vi "+S2C_FORNAX_Process.vi"(8 "Error In":errorcluster) -> (0 "Error Out":errorcluster)   [LabVIEW 2015]
uses:
  VIs/S2C_FORNAX_Proc_Globals.vi
panel:
  out "Err":bool
  out "Init":bool
  in  "Clear":bool
  out "Exit":bool
  in  "LogDepth":u32=500 caption="Log Depth"
  in  "CtrlTab":enum32{"Fornax", "Viper", "DDS Log"}(tab)
  in  "P1":T1 {"P1C1"."Return" items=["Partition", "Message", "M_BarcodeImageFile", "ErrorStatus"]; "P1C1"."Cmd" items=["BarcodeImageCommand", "BoardIdCommand", "Close", "DftAlarmCommand", "DftAudioPlayCommand", "DftInstrumentCommand", "DftLogCommand", "EmA2dCalDataCommand", "EnergyParameterCommand", "ExternalCommCommand", "FeatureSettingsCommand", "FornaxCommand", "General", "InstrumentSettingCommand", "Launch", "MonopolarCommand", "Open", "SupervisorCommand", "SwitchStatus", "SystemConfigurationCommand", "SystemSettingsCommand", "TimeCommand", "UserSettingsCommand", "ViperCmd", "VolumeBarsCommand"]}
  in  "P2":T2={"P2C1"={"VIP_Cmd"="", "VIP_RX"="", "VIP_Browse"=FALSE, "VIP_Send"=FALSE, "VIP_Clear"=FALSE, "VipLogDepth"=50, "VIP_Auto"=TRUE}}
  in  "P3":T3={"P3C1"={"DDS Log"="", "DDS_Clear"=FALSE, "DdsLogDepth"=1000, "DDS_Auto"=TRUE}}
  in  "CommLog":string caption="Communication Log"
  # "Main Cluster:\n394x886\n1 = 355x876\n2 = 355x438\n3 = 355x292\n4 = 163x438\n6 = 163x292\n8 = 163x219"
  # "Fornax Driver Panel"
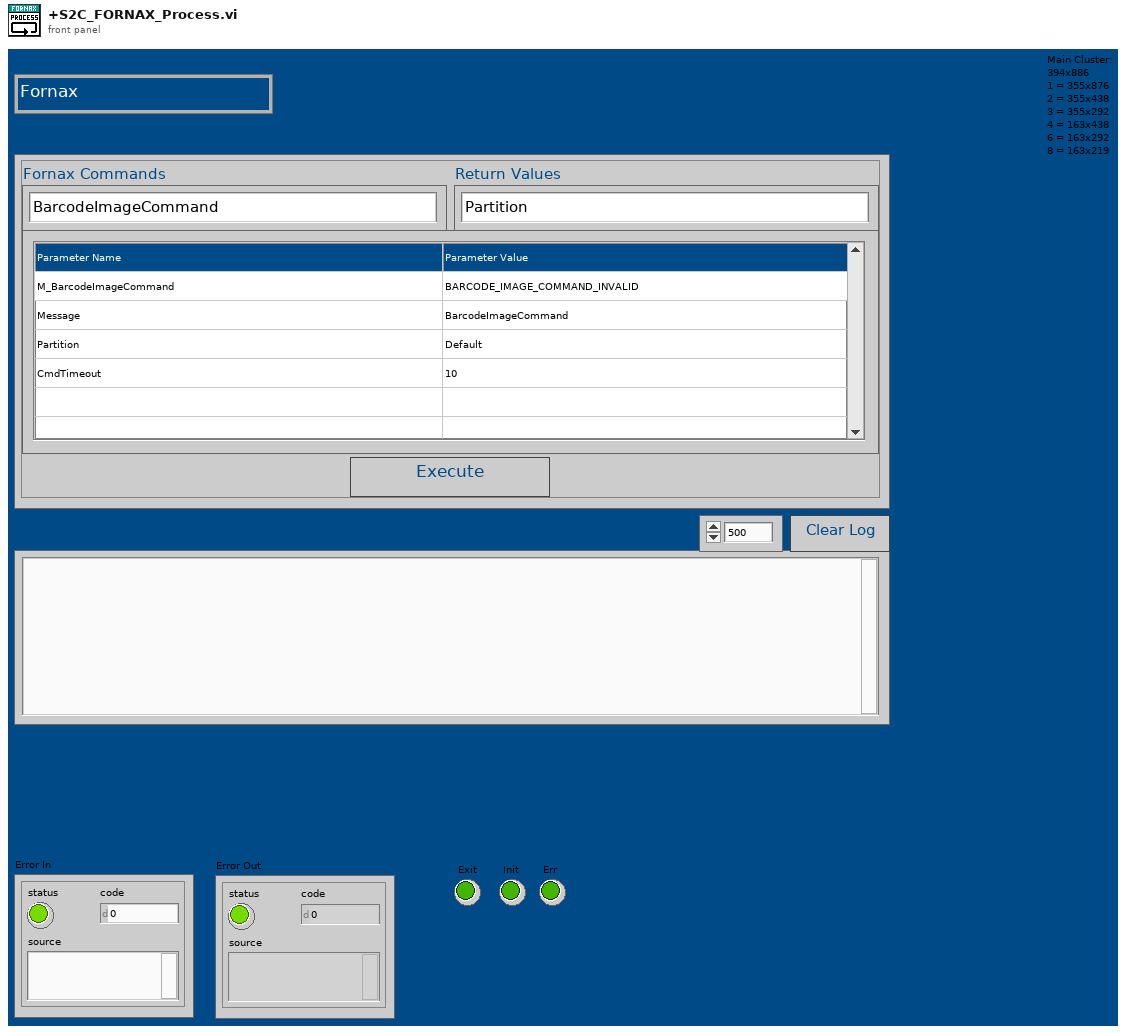
[diagram p1: front panel]
types:
  T1 = cluster{"P1C1":cluster{"P1C1Exe":bool, "Cmd":u16, "Return":u16, "Params":i32}}
  T2 = cluster{"P2C1":cluster{"VIP_Cmd":string, "VIP_RX":string, "VIP_Browse":bool, "VIP_Send":bool, "VIP_Clear":bool, "VipLogDepth":u32, "VIP_Auto":bool}}
  T3 = cluster{"P3C1":cluster{"DDS Log":string, "DDS_Clear":bool, "DdsLogDepth":u32, "DDS_Auto":bool}}
  T4 = cluster{"RawMsg":string, "ViperMsg":string[], "DDSMsg":string[]}
  T5 = typedef "LVPoint32TypeDef.ctl" = cluster{"Horizontal":i32, "Vertical":i32}
  T6 = typedef "LVRowAndColumnTypeDef.ctl" = cluster{"Row":i32, "Column":i32}
  T7 = cluster{"Caller-Q":refnum<queue>, "Command":string, "Return":string, "Data":variant, "Timeout":dbl}
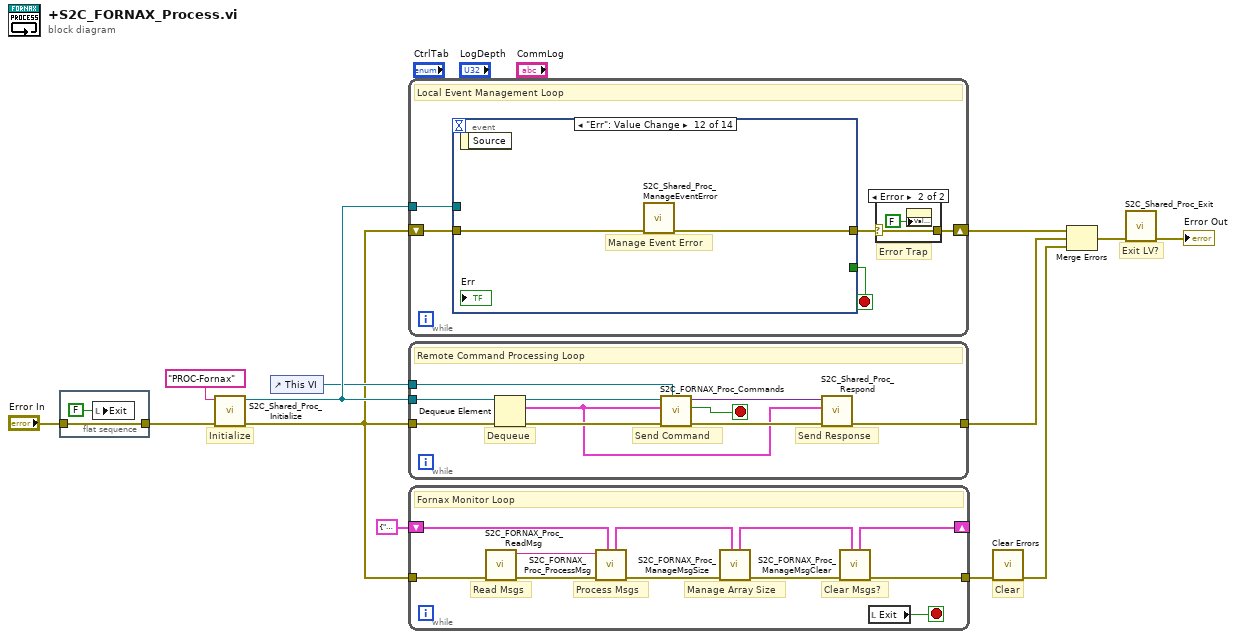
[diagram p0: block diagram]
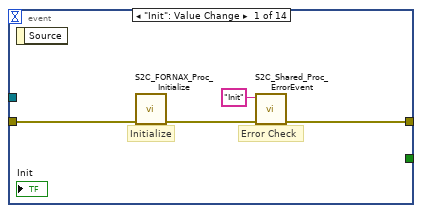
[diagram p3: hidden frame]
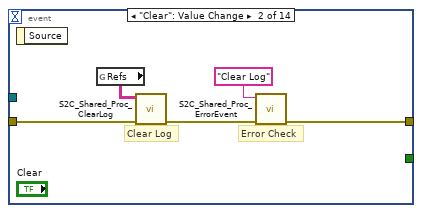
[diagram p4: hidden frame]
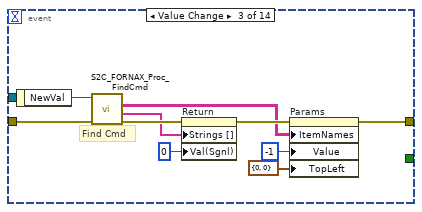
[diagram p5: hidden frame]
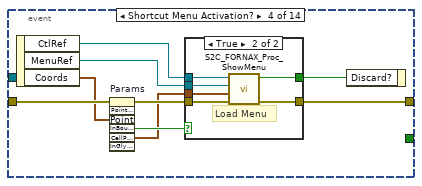
[diagram p6: hidden frame]
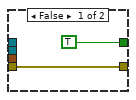
[diagram p7: hidden frame]
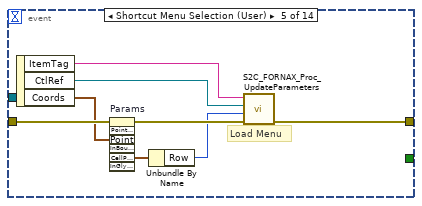
[diagram p8: hidden frame]
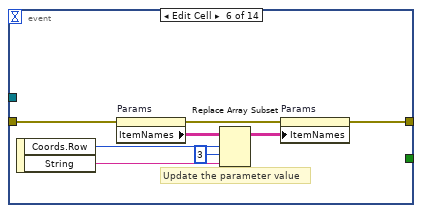
[diagram p9: hidden frame]
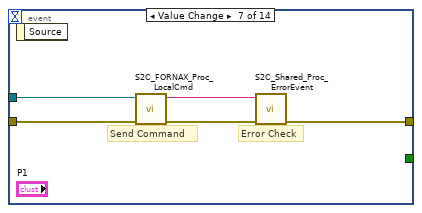
[diagram p10: hidden frame]
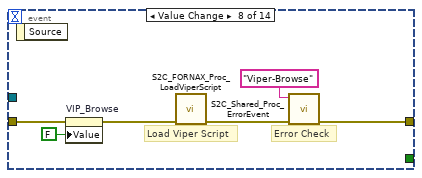
[diagram p11: hidden frame]
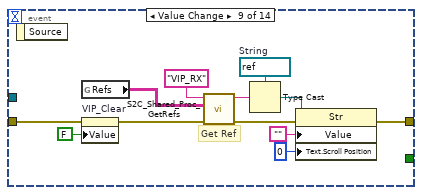
[diagram p12: hidden frame]
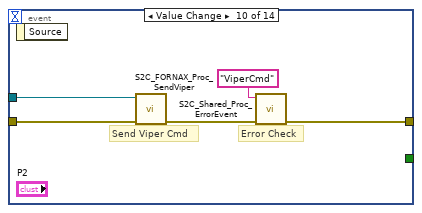
[diagram p13: hidden frame]
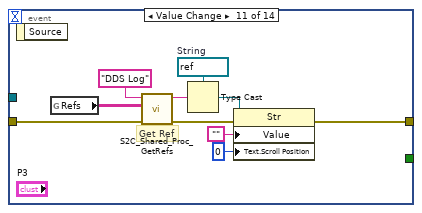
[diagram p14: hidden frame]
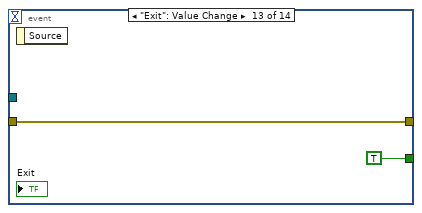
[diagram p15: hidden frame]
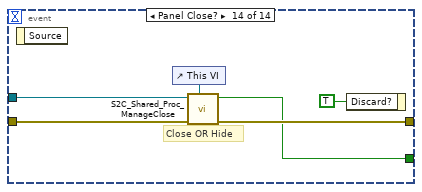
[diagram p16: hidden frame]
diagram:
  # "Clear"
  # "Exit LV?"
  # "Initialize"
  n1 = flat-sequence {
    tunnel: "Error In" -> [w14]
    tunnel: [w14] -> w1
    frame #0 {
      n2 = local write "Exit"(FALSE ("Exit?")) -> ()
    }
  }
  n3 = call "S2C_Shared_Proc_Initialize.vi"("Error In"=w1, "Q-Name"="PROC-Fornax" ("name (unnamed)")) -> ("Error Out"=w2:errorcluster, "Q-Ref"=w9:refnum<queue>)  [unwired: 8 in]
  n4 = control-ref of="This VI"() -> (w6:refnum<vi>)
  n5 = while {
    tunnel: w9 -> [w19]
    shift-right: [w16] -> w13
    shift-left: w2 -> [w20]
    stop <- w18 stop-if-true
    # "Error Trap"
    # "Local Event Management Loop"
    n6 = event shown="[11] \"Err\": Value Change" {
      selector: _ -> [_ _ _ _ _ _ _ _ _ _ _ _ _ _]
      dyn-events: _ -> [_ _ _ _ _ _ _ _ _ _ _ _ _ _]
      timeout: _ -> [_ _ _ _ _ _ _ _ _ _ _ _ _ _]
      tunnel: w20 -> [w27 w32 w42 w51 w67 w75 w79 w86 w89 w103 w106 w115 w117 w122]
      tunnel: w19 -> [_ _ _ _ _ _ w80 _ _ w102 _ _ _ w120]
      tunnel: [w25 w29 w36 w43 w62 w69 w77 w82 w90 w99 w105 w114 w117 w121] -> w17
      tunnel: [_ _ _ _ _ _ _ _ _ _ _ _ TRUE ("Discard?") w119] -> w18
      event "Init": Value Change {
        # "Error Check"
        # "Initialize"
        n7 = event-data() -> ()  [unwired: 1 in, 1 out]
        n8 = call "S2C_FORNAX_Proc_Initialize.vi"("Error In"=w27) -> ("Error Out"=w26:errorcluster)  [unwired: 10 in]
        n9 = call "S2C_Shared_Proc_ErrorEvent.vi"("Error In"=w26, "Command"="Init") -> ("Error Out"=w25:errorcluster)  [unwired: 9 in]
      }
      event "Clear": Value Change {
        # "Error Check"
        # "Clear Log"
        n10 = event-data() -> ()  [unwired: 1 in, 1 out]
        n11 = global read "S2C_FORNAX_Proc_Globals.vi" "Refs"() -> (w31:string[][])
        n12 = call "S2C_Shared_Proc_ClearLog.vi"("Error In"=w32, "Refs"=w31) -> ("Error Out"=w30:errorcluster)  [unwired: 9 in]
        n13 = call "S2C_Shared_Proc_ErrorEvent.vi"("Error In"=w30, "Command"="Clear Log") -> ("Error Out"=w29:errorcluster)  [unwired: 9 in]
      }
      event "P1.P1C1.Cmd": Value Change {
        # "Find Cmd"
        n14 = event-data() -> ("NewVal"=w41:u16)  [unwired: 1 in]
        n15 = call "S2C_FORNAX_Proc_FindCmd.vi"("Error In"=w42, "Index"=w41) -> ("Error Out"=w40:errorcluster, "Returns"=w39:string[], "Parameters"=w33:string[][])  [unwired: 6 in, 1 out]
        n16 = property on="Return" class="Ring (strict)"(error in=w40, "Strings []"=w39, "Val(Sgnl)"=u16 0 ("Value (Signaling)")) -> (error out=w37:errorcluster)  [unwired: 1 in, 1 out]
        n17 = property on="Params" class="MCListbox (strict)"(error in=w37, "ItemNames"=w33, "Value"=-1, "TopLeft"=cluster{"Row":u32, "Column":u32} {"Row"=0, "Column"=0} ("Top Left Visible Cell")) -> (error out=w36:errorcluster)  [unwired: 1 in, 1 out]
      }
      event "P1.P1C1.Params": Shortcut Menu Activation? {
        n18 = event-data() -> ("CtlRef"=w47:refnum<vi>, "MenuRef"=w46:refnum<k9>, "Coords"=w50:T5)  [unwired: 1 in]
        n19 = invoke on="Params" class="MCListbox (strict)" method="Point To Row Column"(error in=w51, "Point"=w50) -> (error out=w49:errorcluster, "InBounds"=w48:bool, "CellPosition"=w45:T6)  [unwired: 5 in, 4 out]
        n20 = case shown="True" w48 {
          tunnel: w49 -> [w53 w59]
          tunnel: w45 -> [_ w58]
          tunnel: w46 -> [_ w57]
          tunnel: w47 -> [_ w56]
          tunnel: [w53 w55] -> w43
          tunnel: [TRUE ("Discard?") w54] -> w44
          frame False {
          }
          frame True {
            # "Load Menu"
            n21 = call "S2C_FORNAX_Proc_ShowMenu.vi"("Error In"=w59, "Cell Position"=w58, "MenuRef"=w57, "CtlRef"=w56) -> ("Error Out"=w55:errorcluster, "Discard?"=w54:bool)  [unwired: 6 in]
          }
        }
        n22 = event-data("Discard?"=w44) -> ()  [unwired: 1 in, 1 out]
      }
      event "P1.P1C1.Params": Shortcut Menu Selection (User) {
        # "Load Menu"
        n23 = event-data() -> ("ItemTag"=w64:string, "CtlRef"=w63:refnum<vi>, "Coords"=w66:T5)  [unwired: 1 in]
        n24 = invoke on="Params" class="MCListbox (strict)" method="Point To Row Column"(error in=w67, "Point"=w66) -> (error out=w65:errorcluster, "CellPosition"=w61:T6)  [unwired: 5 in, 5 out]
        n25 = Unbundle By Name(w61) -> ("Row"=w60:i32)
        n26 = call "S2C_FORNAX_Proc_UpdateParameters.vi"("Error In"=w65, "Row"=w60, "CtlRef"=w63, "ItemTag"=w64) -> ("Error Out"=w62:errorcluster)  [unwired: 7 in]
      }
      event "P1.P1C1.Params": Edit Cell {
        # "Update the parameter value"
        n27 = event-data() -> ("Coords.Row"=w71:i32, "String"=w72:string)  [unwired: 1 in]
        n28 = property on="Params" class="MCListbox (strict)"(error in=w75) -> (error out=w70:errorcluster, "ItemNames"=w73:string[][])  [unwired: 1 in, 1 out]
        n29 = Replace Array Subset(array=w73, new element=w72, index (row)=w71, index (col)=3 ("disabled index (col)")) -> (w68:string[][])
        n30 = property on="Params" class="MCListbox (strict)"(error in=w70, "ItemNames"=w68) -> (error out=w69:errorcluster)  [unwired: 1 in, 1 out]
      }
      event "P1.P1C1.P1C1Exe": Value Change {
        # "Error Check"
        # "Send Command"
        n31 = event-data() -> ()  [unwired: 1 in, 1 out]
        n32 = call "S2C_FORNAX_Proc_LocalCmd.vi"("Error In"=w79, "Q-Ref"=w80) -> ("Error Out"=w78:errorcluster, "Command"=w76:string)  [unwired: 8 in]
        n33 = call "S2C_Shared_Proc_ErrorEvent.vi"("Error In"=w78, "Command"=w76) -> ("Error Out"=w77:errorcluster)  [unwired: 9 in]
      }
      event "P2.P2C1.VIP_Browse": Value Change {
        # "Error Check"
        # "Load Viper Script"
        n34 = event-data() -> ()  [unwired: 1 in, 1 out]
        n35 = property on="VIP_Browse" class="Bool (strict)"(error in=w86, "Value"=FALSE) -> (error out=w85:errorcluster)  [unwired: 1 in, 1 out]
        n36 = call "S2C_FORNAX_Proc_LoadViperScript.vi"("Error In"=w85) -> ("Error Out"=w83:errorcluster)  [unwired: 10 in]
        n37 = call "S2C_Shared_Proc_ErrorEvent.vi"("Error In"=w83, "Command"="Viper-Browse") -> ("Error Out"=w82:errorcluster)  [unwired: 9 in]
      }
      event "P2.P2C1.VIP_Clear": Value Change {
        w96 = refnum<vi> refnum  # String
        # "Get Ref"
        n38 = event-data() -> ()  [unwired: 1 in, 1 out]
        n39 = global read "S2C_FORNAX_Proc_Globals.vi" "Refs"() -> (w91:string[][])
        n40 = property on="VIP_Clear" class="Bool (strict)"(error in=w89, "Value"=FALSE) -> (error out=w88:errorcluster)  [unwired: 1 in, 1 out]
        n41 = call "S2C_Shared_Proc_GetRefs.vi"("Error In"=w88, "Refs"=w91, "Label"="VIP_RX") -> ("Error Out"=w95:errorcluster, "Reference"=w97:string)  [unwired: 7 in]
        n42 = Type Cast(type=w96, x=w97) -> (*(type *) &x=w98:refnum<vi>)
        n43 = property class="Str"(reference=w98, error in=w95, "Value"="", "Text.Scroll Position"=u32 0) -> (error out=w90:errorcluster)  [unwired: 1 out]
      }
      event "P2.P2C1.VIP_Send": Value Change {
        # "Error Check"
        # "Send Viper Cmd"
        n44 = event-data() -> ()  [unwired: 1 in, 1 out]
        n45 = call "S2C_FORNAX_Proc_SendViper.vi"("Error In"=w103, "Q-Ref"=w102) -> ("Error Out"=w101:errorcluster)  [unwired: 9 in]
        n46 = call "S2C_Shared_Proc_ErrorEvent.vi"("Error In"=w101, "Command"="ViperCmd") -> ("Error Out"=w99:errorcluster)  [unwired: 9 in]
      }
      event "P3.P3C1.DDS_Clear": Value Change {
        w111 = refnum<vi> refnum  # String
        # "Get Ref"
        n47 = event-data() -> ()  [unwired: 1 in, 1 out]
        n48 = global read "S2C_FORNAX_Proc_Globals.vi" "Refs"() -> (w104:string[][])
        n49 = call "S2C_Shared_Proc_GetRefs.vi"("Error In"=w106, "Refs"=w104, "Label"="DDS Log") -> ("Error Out"=w110:errorcluster, "Reference"=w112:string)  [unwired: 7 in]
        n50 = Type Cast(type=w111, x=w112) -> (*(type *) &x=w113:refnum<vi>)
        n51 = property class="Str"(reference=w113, error in=w110, "Value"="", "Text.Scroll Position"=u32 0) -> (error out=w105:errorcluster)  [unwired: 1 out]
      }
      event "Err": Value Change {
        # "Manage Event Error"
        n52 = event-data() -> ()  [unwired: 1 in, 1 out]
        n53 = call "S2C_Shared_Proc_ManageEventError.vi"("Error In"=w115) -> ("Error Out"=w114:errorcluster)  [unwired: 10 in]
      }
      event "Exit": Value Change {
        n54 = event-data() -> ()  [unwired: 1 in, 1 out]
      }
      event Panel Close? {
        # "Close OR Hide"
        n55 = event-data() -> ()  [unwired: 1 in, 1 out]
        n56 = control-ref of="This VI"() -> (w118:refnum<vi>)
        n57 = call "S2C_Shared_Proc_ManageClose.vi"("VI_Ref"=w118, "Error In"=w122, "Q-Ref"=w120) -> ("Error Out"=w121:errorcluster, "Exit?"=w119:bool)  [unwired: 7 in]
        n58 = event-data("Discard?"=TRUE) -> ()  [unwired: 1 in, 1 out]
      }
    }
    n59 = case shown="Error" w17 {
      selector: w17 -> [w21 w23]
      tunnel: [w21 w23] -> w16
      frame No Error {
      }
      frame Error {
        n60 = property on="Err" class="Bool (strict)"("Val(Sgnl)"=FALSE ("Value (Signaling)")) -> ()  [unwired: 2 in, 2 out]
      }
    }
  }
  n61 = while {
    tunnel: w9 -> [w132]
    tunnel: w2 -> [w133]
    tunnel: [w128] -> w8
    tunnel: w6 -> [w127]
    stop <- w126 stop-if-true
    # "Send Command"
    # "Send Response"
    # "Dequeue"
    # "Remote Command Processing Loop"
    n62 = Dequeue Element(queue=w132, error in (no error)=w133) -> (queue out=w125:refnum<queue>, element=w124:T7, error out=w131:errorcluster)  [unwired: 1 in, 1 out]
    n63 = call "S2C_FORNAX_Proc_Commands.vi"("VI_Ref"=w127, "Error In"=w131, "Settings"=w124, "Q-Ref"=w125) -> ("Error Out"=w129:errorcluster, "Exit?"=w126:bool, "Response"=w130:variant)  [unwired: 5 in]
    n64 = call "S2C_Shared_Proc_Respond.vi"("Error In"=w129, "Settings"=w124, "Response"=w130) -> ("Error Out"=w128:errorcluster)  [unwired: 8 in]
  }
  n65 = while {
    tunnel: w2 -> [w144]
    shift-right: [w135] -> _
    shift-left: T4 {"RawMsg"="", "ViperMsg"=[], "DDSMsg"=[]} -> [w134]
    tunnel: [w136] -> w7
    stop <- w143 stop-if-true
    # "Clear Msgs?"
    # "Manage Array Size"
    # "Process Msgs"
    # "Read Msgs"
    # "Fornax Monitor Loop"
    n66 = call "S2C_FORNAX_Proc_ReadMsg.vi"("Error In"=w144) -> ("Error Out"=w142:errorcluster, "Message"=w140:string)  [unwired: 9 in]
    n67 = call "S2C_FORNAX_Proc_ProcessMsg.vi"("Msg In"=w134, "Error In"=w142, "Message"=w140) -> ("Error Out"=w141:errorcluster, "Msg Out"=w139:T4)  [unwired: 7 in]
    n68 = call "S2C_FORNAX_Proc_ManageMsgSize.vi"("Msg In"=w139, "Error In"=w141) -> ("Error Out"=w138:errorcluster, "Msg Out"=w137:T4)  [unwired: 8 in]
    n69 = call "S2C_FORNAX_Proc_ManageMsgClear.vi"("Msg In"=w137, "Error In"=w138) -> ("Error Out"=w136:errorcluster, "Msg Out"=w135:T4)  [unwired: 8 in]
    n70 = local read "Exit"() -> (w143:bool)
  }
  n71 = call <vilib>:"Clear Errors.vi"("error in (no error)"=w7) -> ("error out"=w3:errorcluster)  [unwired: 5 in, 1 out]
  n72 = Merge Errors(w13, w8, w3) -> (w5:errorcluster)
  n73 = call "S2C_Shared_Proc_Exit.vi"("Error In"=w5) -> ("Error Out"=→"Error Out":errorcluster)  [unwired: 10 in]
